vi "LAOnFunctionCall.vi"(8 "Error In":errorcluster, 11 "LiteAgent In":T2) -> (0 "Error Out":errorcluster, 1 "FunctionCall":T1, 2 "SessionId":string, 3 "LiteAgent Out":T2)   [LabVIEW 2017, in "LiteAgentSDK.lvlib"]
uses:
  LiteAgentSDK.lvlib
  C:/Users/Jan/Projects/LiteAgentSDK-LabVIEW/Source/Bin/LiteAgentSDK.LabVIEW.dll
  Bin/LiteAgentSDK.LabVIEW.dll
  <vilib>/LVH/i3 JSON/JSON Parsing/Get Object Parameter Files/Get Object Parameter - String.vi
  <vilib>/LVH/i3 JSON/JSON Parsing/Get Object Parameter Files/Get Object Parameter - Object.vi
  <vilib>/LVH/i3 JSON/i3-json.lvlib
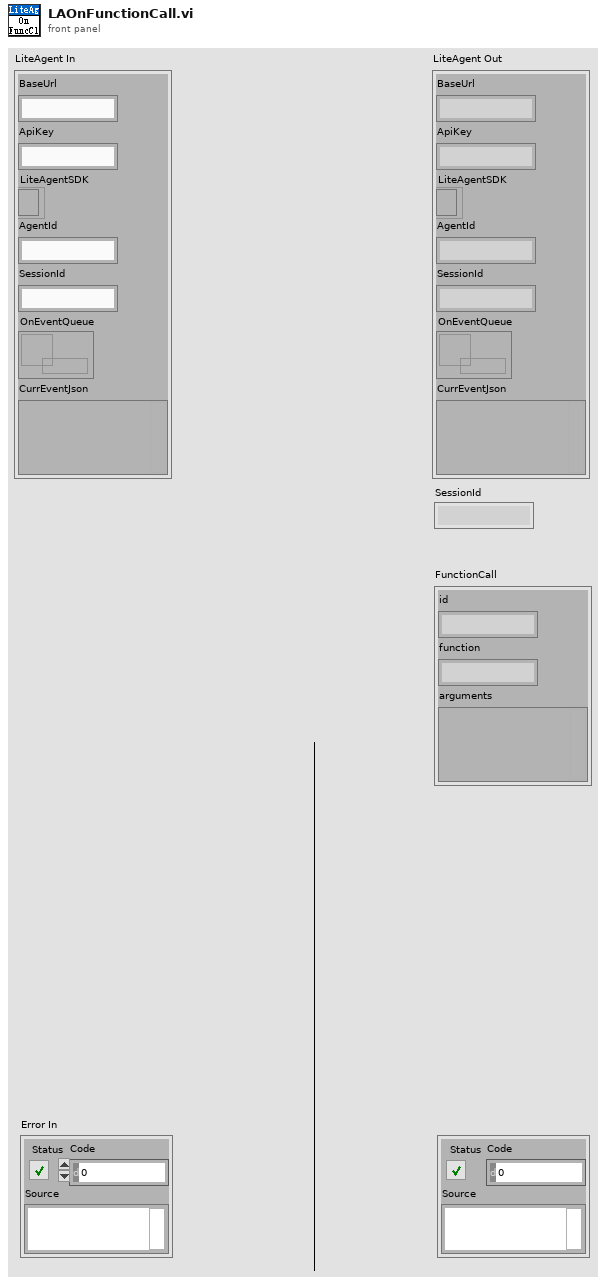
[diagram p1: front panel]
types:
  T1 = cluster{"id":string, "function":string, "arguments":variant}
  T2 = cluster{"BaseUrl":string, "ApiKey":string, "LiteAgentSDK":refnum<k24>, "AgentId":string, "SessionId":string, "OnEventQueue":refnum<queue>, "CurrEventJson":variant}
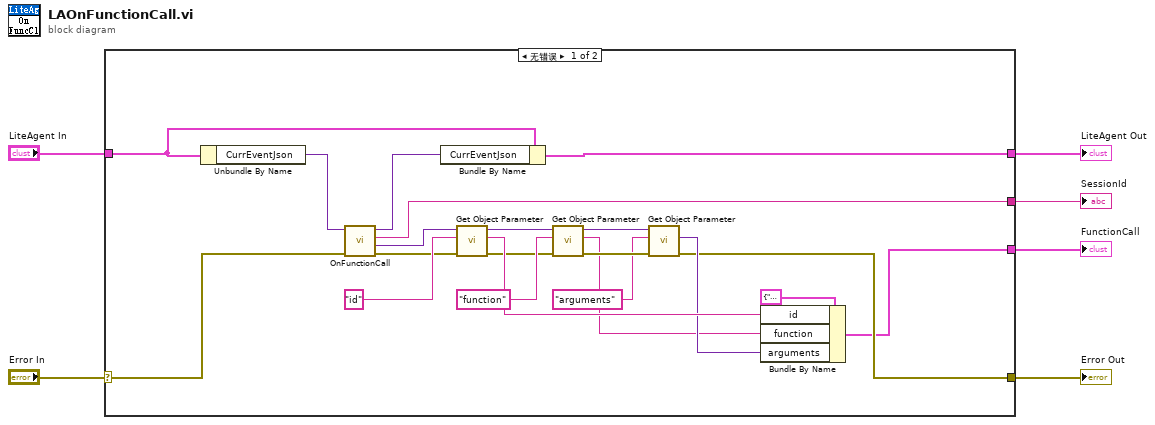
[diagram p0: block diagram]
diagram:
  n1 = case shown="无错误" "Error In" {
    selector: "Error In" -> [w24 w29]
    tunnel: [w10 w29] -> w5
    tunnel: "LiteAgent In" -> [w27 w28]
    tunnel: [w26 w28] -> w3
    tunnel: [w16 _] -> w2
    tunnel: [w8 _] -> w1
    frame No Error {
      n2 = Unbundle By Name(w27) -> ("CurrEventJson"=w25:variant)
      n3 = call "OnFunctionCall.vi"("Error In"=w24, "JSON Tree In"=w25) -> ("Error Out"=w11:errorcluster, "Payload"=w17:variant, "SessionId"=w16:string, "JSON Tree Out"=w23:variant)  [unwired: 6 in]
      n4 = Bundle By Name(cluster=w27, "CurrEventJson"=w23) -> (w26:T2)
      n5 = call-poly <vilib>:"Get Object Parameter.vi"("error in (no error)"=w11, "Parameter Name"="id", "JSON Tree In (JSON Object)"=w17) -> ("error out"=w9:errorcluster, "String Value"=w13:string, "JSON Tree Out Passthrough"=w22:variant)  [unwired: 5 in, 1 out]
      n6 = call-poly <vilib>:"Get Object Parameter.vi"("error in (no error)"=w9, "Parameter Name"="function", "JSON Tree In (JSON Object)"=w22) -> ("error out"=w20:errorcluster, "String Value"=w7:string, "JSON Tree Out Passthrough"=w21:variant)  [unwired: 5 in, 1 out]
      n7 = call-poly <vilib>:"Get Object Parameter.vi"("error in (no error)"=w20, "Parameter Name"="arguments", "JSON Tree In (JSON Object)"=w21) -> ("error out"=w10:errorcluster, "JSON Object"=w12:variant)  [unwired: 5 in, 2 out]
      n8 = Bundle By Name(cluster=T1 {"id"="", "function"="", "arguments"=variant} ("FunctionCall"), "id"=w13, "function"=w7, "arguments"=w12) -> (w8:T1)
    }
    frame Error {
    }
  }
  "Error Out" <- w5
  "LiteAgent Out" <- w3
  "SessionId" <- w2
  "FunctionCall" <- w1
